vi "RichToFlatrfcontrol_SetTriggerWaitResponse.vi"(5 "OutputClusterType":T1, 11 "InputCluster":T2) -> (3 "OutputCluster":T1)   [LabVIEW 2024, in "FlexSDR_gRPC_client.lvlib"]
uses:
  rfcontrol_SetTriggerWaitResponse.ctl
  rfcontrol_SetTriggerWaitResponse_Flat.ctl
  FlexSDR_gRPC_client.lvlib
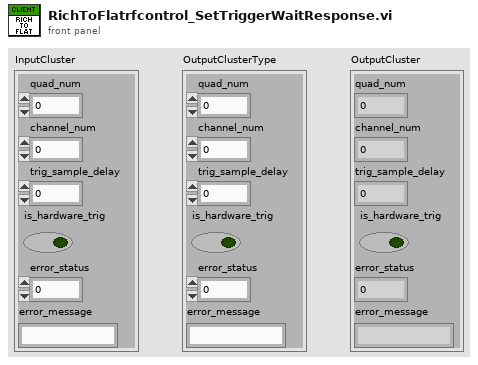
[diagram p1: front panel]
types:
  T1 = typedef "FlexSDR_gRPC_client.lvlib/rfcontrol_SetTriggerWaitResponse_Flat.ctl" = cluster{"quad_num":i32, "channel_num":i32, "trig_sample_delay":i32, "is_hardware_trig":bool, "error_status":i32, "error_message":string}
  T2 = typedef "FlexSDR_gRPC_client.lvlib/rfcontrol_SetTriggerWaitResponse.ctl" = cluster{"quad_num":i32, "channel_num":i32, "trig_sample_delay":i32, "is_hardware_trig":bool, "error_status":i32, "error_message":string}
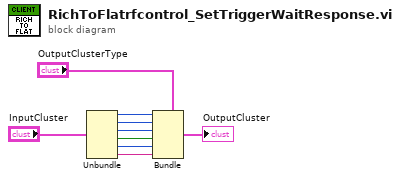
[diagram p0: block diagram]
diagram:
  n1 = Unbundle "Unbundle"("InputCluster") -> ("quad_num"=w6:i32, "channel_num"=w5:i32, "trig_sample_delay"=w4:i32, "is_hardware_trig"=w3:bool, "error_status"=w2:i32, "error_message"=w1:string)
  n2 = Bundle "Bundle"(cluster="OutputClusterType", "quad_num"=w6, "channel_num"=w5, "trig_sample_delay"=w4, "is_hardware_trig"=w3, "error_status"=w2, "error_message"=w1) -> (→"OutputCluster":T1)
